vi "CommonVIs_UpdateAttributeCtrlPath.vi"(9 "Class/TypePath":path[](array[path]), 10 "Class/TypeName":string[](array[string]), 11 "DataType in":T1) -> (3 "DataType out":T1)   [LabVIEW 2012]
uses:
  <resource>/Framework/Providers/Open_GDS/ClassProviders/Common/CommonVIs/CommonVIs_AttributeType.ctl
  <resource>/Framework/Providers/Open_GDS/ClassProviders/Common/CommonVIs/CommonVIs_AttributeDataType.ctl
  <resource>/Framework/Providers/Open_GDS/ClassProviders/Common/String/GDSString_AccessScopeModifierType.ctl
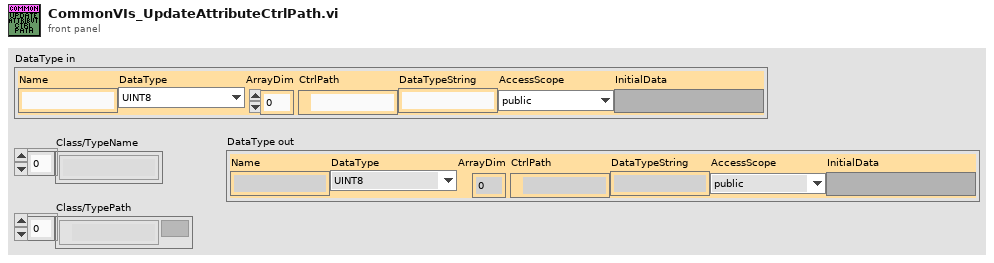
[diagram p1: front panel]
types:
  T1 = typedef "CommonVIs_AttributeType.ctl" = cluster{"Name":string, "DataType":T2, "ArrayDim":i32, "CtrlPath":path, "DataTypeString":string, "AccessScope":T3, "InitialData":variant}
  T2 = typedef "CommonVIs_AttributeDataType.ctl" = enum16{"UINT8", "INT8", "UINT16", "INT16", "UINT32", "INT32", "UINT64", "INT64", "SGL", "DBL", "EXT", "CSG", "CDB", "CXT", "TimeStamp", "STRING", "PATH", "BOOL", "ENUM", "RefNum", "VIRefNum", "LabVIEW Class", "Cluster", "Variant", "TypeDef", "Waveform", "LabVIEW Object", "Other", "void"}
  T3 = typedef "GDSString_AccessScopeModifierType.ctl" = enum16{"public", "private", "protected", "internal"}
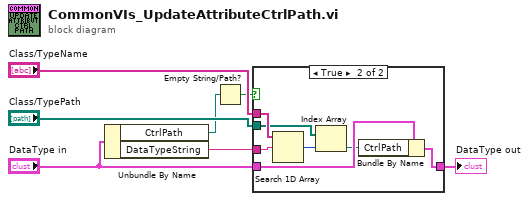
[diagram p0: block diagram]
diagram:
  n1 = Unbundle By Name("DataType in") -> ("CtrlPath"=w1:path, "DataTypeString"=w3:string)
  n2 = Empty String/Path?(string/path=w1) -> (empty?=w2:bool)
  n3 = case shown="True" w2 {
    tunnel: w3 -> [_ w15]
    tunnel: "Class/TypeName" -> [_ w14]
    tunnel: "Class/TypePath" -> [_ w12]
    tunnel: "DataType in" -> [w8 w11]
    tunnel: [w8 w10] -> w7
    frame False {
    }
    frame True {
      n4 = Search 1D Array(1D array=w14, element=w15) -> (index of element=w13:i32)  [unwired: 1 in]
      n5 = Index Array(array=w12, index=w13) -> (element=w9:path)
      n6 = Bundle By Name(cluster=w11, "CtrlPath"=w9) -> (w10:T1)
    }
  }
  "DataType out" <- w7
